vi "主界面.vi"() -> ()   [LabVIEW 2016]
uses:
  <vilib>/Hampel Software Engineering/HSE Logger/LogLevel.ctl
  <vilib>/Utility/miscctls.llb/LVPointTypeDef.ctl
  <vilib>/picture/picture.llb/imagedata.ctl
  <vilib>/Hampel Software Engineering/HSE Logger/Handler/FileHandler/FileHandler.lvclass
  C:/Program Files (x86)/National Instruments/LabVIEW 2016/vi.lib/Hampel Software Engineering/HSE Logger/Handler/Handler.lvclass
  <vilib>/Utility/config.llb/NI_LVConfig.lvlib
  <vilib>/Utility/LVLibp/NI_PackedLibraryUtility.lvlib
  update/update.lvlib
  <vilib>/Hampel Software Engineering/HSE Logger/hse-logger.lvlib
panel:
  in  "删除按钮":bool
  in  "添加按钮":bool
  in  "单选按钮":T1(radio)=enum."单选选项2"
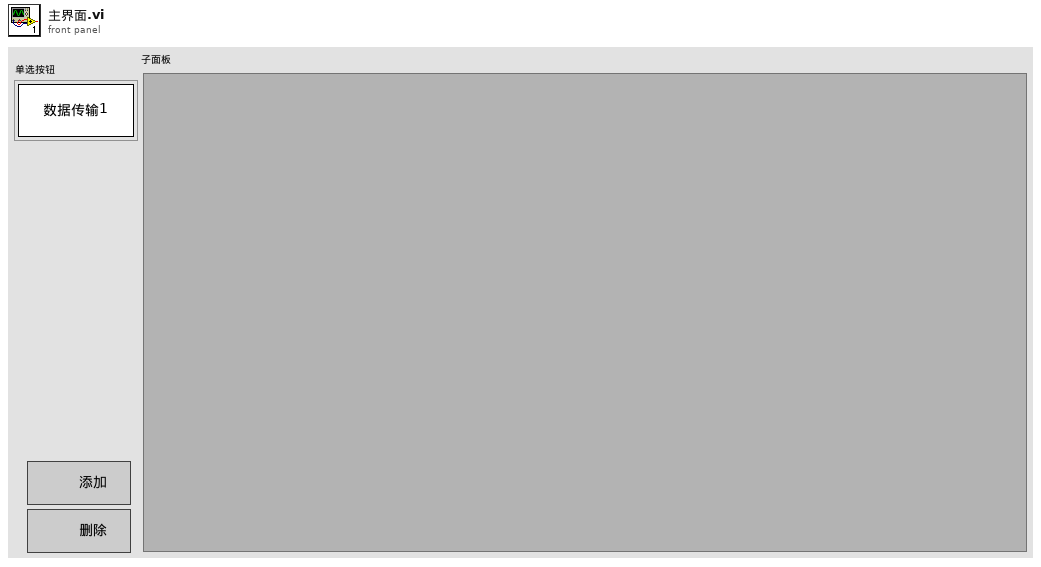
[diagram p1: front panel]
types:
  T1 = enum32{"数据传输1", "单选选项2", "单选选项3", "单选选项4", "单选选项5", "单选选项6"}
  T2 = typedef "hse-logger.lvlib/LogLevel.ctl" = enum16{"DEBUG", "INFO", "WARNING", "ERROR", "CRITICAL"}
  T3 = typedef "imagedata.ctl" = cluster{"image type":i32, "image depth":i32, "image":u8[], "mask":u8[], "colors":u32[], "Rectangle":cluster{"left":i16, "top":i16, "right":i16, "bottom":i16}}
  T4 = typedef "LVPointTypeDef.ctl" = cluster{"Horizontal":i16, "Vertical":i16}
  T5 = typedef "NI_LVConfig.lvlib/Config Data RefNum.ctl" = refnum<k1>
  T6 = enum32{"Bad", "Idle", "Run top level", "Running"}
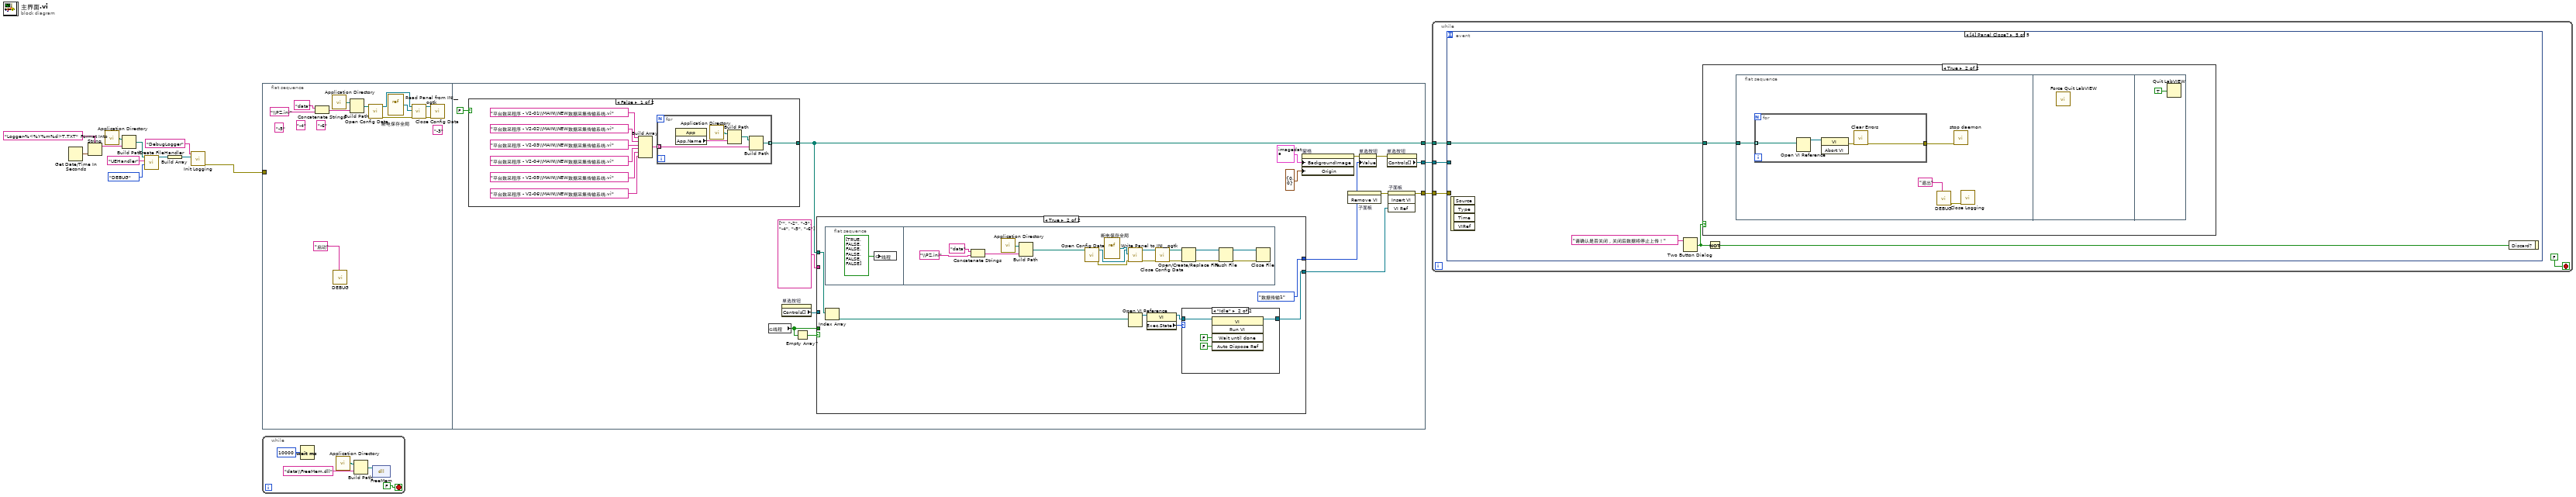
[diagram p0: block diagram]
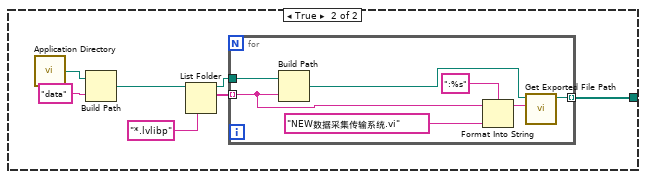
[diagram p2: hidden frame]
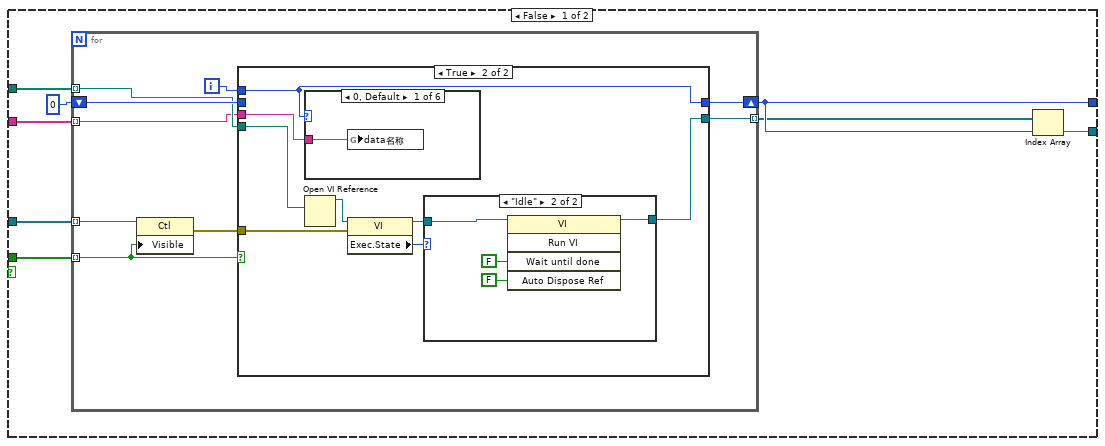
[diagram p3: hidden frame]
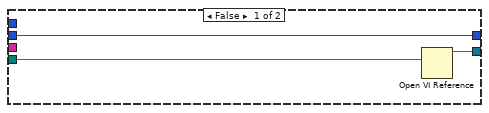
[diagram p4: hidden frame]
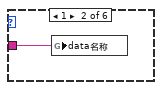
[diagram p5: hidden frame]
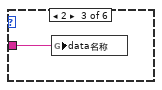
[diagram p6: hidden frame]
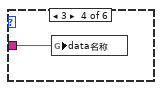
[diagram p7: hidden frame]
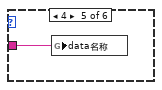
[diagram p8: hidden frame]
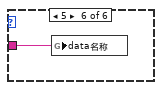
[diagram p9: hidden frame]
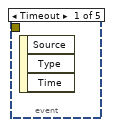
[diagram p12: hidden frame]
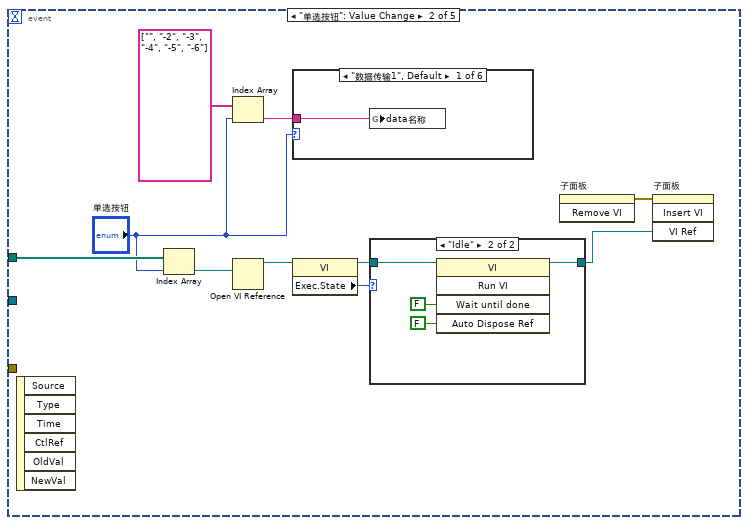
[diagram p13: hidden frame]
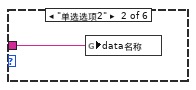
[diagram p14: hidden frame]
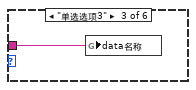
[diagram p15: hidden frame]
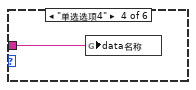
[diagram p16: hidden frame]
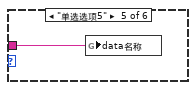
[diagram p17: hidden frame]
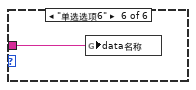
[diagram p18: hidden frame]
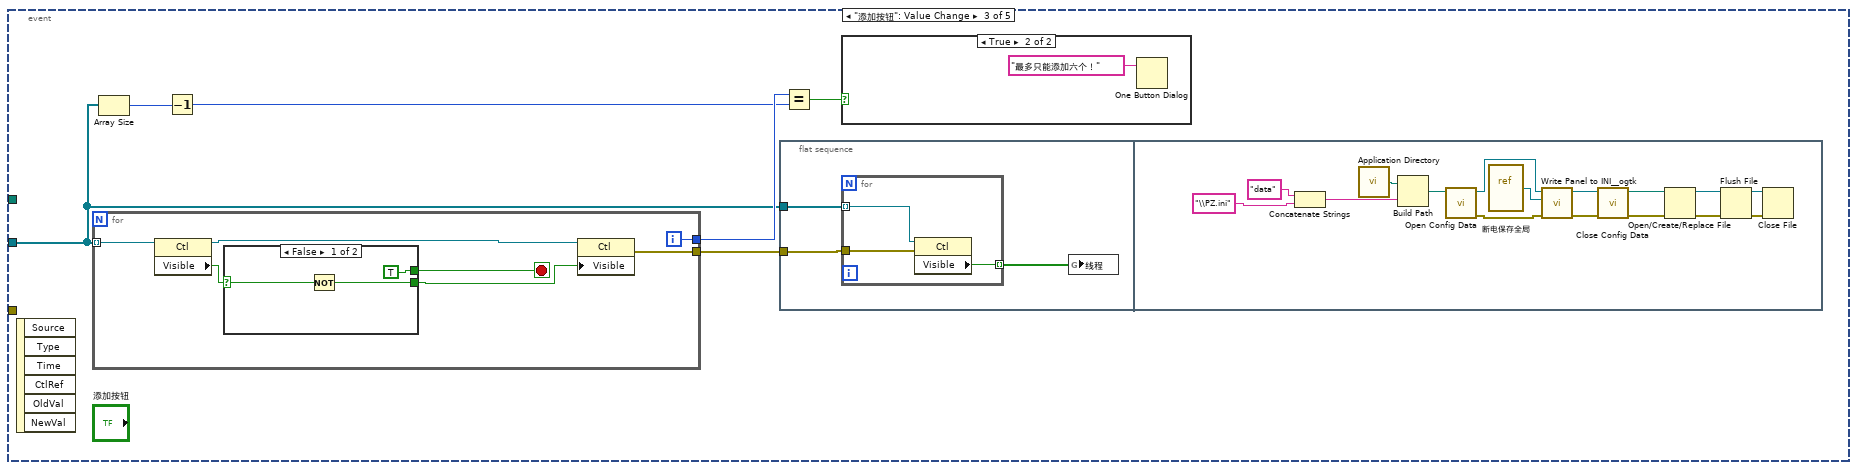
[diagram p20: hidden frame]
diagram:
  n1 = Get Date/Time In Seconds() -> (seconds since 1Jan1904=w4:timestamp)
  n2 = Format Into String(format string="Logger-%<%Y%m%d>T.TXT", w4) -> (resulting string=w5:string)  [unwired: 2 in, 1 out]
  n3 = call <vilib>:"Application Directory.vi"() -> ("Application Directory"=w7:path)
  n4 = Build Path(base path=w7, name or relative path=w5) -> (appended path=w6:path)
  n5 = call <vilib>:"Create FileHandler.vi"("Level"=LogLevel."DEBUG", "Name"="UEHandler", "Filepath"=w6) -> ("FileHandler out"=w9:refnum<class "FileHandler.lvclass">)  [unwired: 7 in, 1 out]
  n6 = Build Array(w9) -> (w10:refnum<class "FileHandler.lvclass">[])
  n7 = call <vilib>:"Init Logging.vi"("Handlers"=w10, "Name"="DebugLogger") -> ("error out"=w1:errorcluster)  [unwired: 9 in]
  n8 = flat-sequence {
    tunnel: w1 -> [_]
    tunnel: [w39] -> w14
    tunnel: [w38] -> w13
    tunnel: [w28] -> w12
    frame #0 {
      (unwired) "-6" ("data名称")
      (unwired) "-5" ("data名称")
      (unwired) "-4" ("data名称")
      (unwired) "-3" ("data名称")
      n9 = Concatenate Strings("data" ("名称或相对路径"), "\\PZ.ini" ("名称或相对路径")) -> (w24:string)
      n10 = call <vilib>:"Application Directory.vi"() -> ("Application Directory"=w20:path)
      n11 = call <vilib>:"DEBUG.vi"("Message"="启动") -> ()  [unwired: 10 in, 1 out]
      n12 = Build Path(base path=w20, name or relative path=w24) -> (appended path=w21:path)
      n13 = call <vilib>:"Open Config Data.vi"("configuration file path"=w21) -> ("error out"=w16:errorcluster, "refnum"=w17:T5)  [unwired: 8 in, 1 out]
      n14 = vi-ref "断电保存全局.vi"() -> (w18:refnum<vi>)
      n15 = call <userlib>:"Read Panel from INI__ogtk.vi"("error in (no error)"=w16, "VI ref"=w18, "refnum"=w17) -> ("error out"=w22:errorcluster, "refnum out"=w19:T5)  [unwired: 7 in]
      n16 = call <vilib>:"Close Config Data.vi"("error in (no error)"=w22, "refnum"=w19) -> ()  [unwired: 8 in, 2 out]
    }
    frame #1 {
      n17 = case shown="False" FALSE {
        tunnel: [w41 w54] -> w28
        frame False {
          n18 = Build Array("平台数采程序 - V2-01\\MAIN\\NEW数据采集传输系统.vi" ("名称或相对路径"), "平台数采程序 - V2-02\\MAIN\\NEW数据采集传输系统.vi" ("名称或相对路径"), "平台数采程序 - V2-03\\MAIN\\NEW数据采集传输系统.vi" ("名称或相对路径"), "平台数采程序 - V2-04\\MAIN\\NEW数据采集传输系统.vi" ("名称或相对路径"), "平台数采程序 - V2-05\\MAIN\\NEW数据采集传输系统.vi" ("名称或相对路径"), "平台数采程序 - V2-06\\MAIN\\NEW数据采集传输系统.vi" ("名称或相对路径")) -> (w48:string[])
          n19 = for {
            tunnel: w48 -> [w53] mode=indexing
            tunnel: [w52] -> w41 mode=indexing
            n20 = property class="App"() -> ("App.Name"=w51:string)  [unwired: 2 in, 2 out]
            n21 = call <vilib>:"Application Directory.vi"() -> ("Application Directory"=w50:path)
            n22 = Build Path(base path=w50, name or relative path=w51) -> (appended path=w49:path)
            n23 = Build Path(base path=w49, name or relative path=w53) -> (appended path=w52:path)
          }
        }
        frame True {
          n24 = call <vilib>:"Application Directory.vi"() -> ("Application Directory"=w57:path)
          n25 = Build Path(base path=w57, name or relative path="data" ("名称或相对路径")) -> (appended path=w59:path)
          n26 = List Folder(path=w59, pattern="*.lvlibp" ("类型")) -> (path out=w55:path, filenames=w56:string[])  [unwired: 2 in, 2 out]
          n27 = for {
            tunnel: w55 -> [w67]
            tunnel: w56 -> [w64] mode=indexing
            tunnel: [w61] -> w54 mode=indexing
            n28 = Build Path(base path=w67, name or relative path=w64) -> (appended path=w63:path)
            n29 = Format Into String(format string=":%s" ("格式字符串"), initial string=w64, "NEW数据采集传输系统.vi" ("输入 1")) -> (resulting string=w62:string)  [unwired: 1 in, 1 out]
            n30 = call <vilib>:"Get Exported File Path.vi"("qualified name"=w62, "packed library path"=w63) -> ("path"=w61:path)  [unwired: 8 in, 1 out]
          }
        }
      }
      n31 = global read "断电保存全局.vi" "线程"() -> (w33:bool[])
      n32 = property on="单选按钮" class="RadioBtnsControl (strict)"() -> ("Controls[]"=w32:refnum<vi>[])  [unwired: 2 in, 2 out]
      n33 = Empty Array?(array=w33) -> (empty?=w34:bool)
      n34 = case shown="True" w34 {
        tunnel: [w73 w111] -> w31
        tunnel: w33 -> [w75 _]
        tunnel: w32 -> [w74 _]
        tunnel: [w71 T1."数据传输1" ("单选按钮")] -> w30
        tunnel: w28 -> [w69 w108]
        tunnel: string[] ["", "-2", "-3", "-4", "-5", "-6"] -> [w68 _]
        frame False {
          n35 = for {
            tunnel: [w84] -> w70 mode=indexing
            tunnel: w75 -> [w83] mode=indexing
            tunnel: w74 -> [w82] mode=indexing
            shift-right: [w79] -> w71
            shift-left: 0 -> [w78]
            tunnel: w69 -> [w77] mode=indexing
            tunnel: w68 -> [w76] mode=indexing
            i -> [w80]
            n36 = property class="Ctl"(reference=w82, "Visible"=w83) -> (error out=w81:errorcluster)  [unwired: 1 in, 1 out]
            n37 = case shown="True" w83 {
              tunnel: [w86 w93] -> w84
              tunnel: w81 -> [_ w92]
              tunnel: w80 -> [_ w89]
              tunnel: [w87 w89] -> w79
              tunnel: w78 -> [w87 _]
              tunnel: w77 -> [w85 w90]
              tunnel: w76 -> [_ w88]
              frame False {
                n38 = Open VI Reference(vi path=w85) -> (vi reference=w86:refnum<vi>)  [unwired: 5 in, 1 out]
              }
              frame True {
                n39 = case shown="0, Default" w89 {
                  tunnel: w88 -> [w96 w97 w98 w99 w100 w101]
                  frame 0, Default {
                    n40 = global write "断电保存全局.vi" "data名称"(w96) -> ()
                  }
                  frame 1 {
                    n41 = global write "断电保存全局.vi" "data名称"(w97) -> ()
                  }
                  frame 2 {
                    n42 = global write "断电保存全局.vi" "data名称"(w98) -> ()
                  }
                  frame 3 {
                    n43 = global write "断电保存全局.vi" "data名称"(w99) -> ()
                  }
                  frame 4 {
                    n44 = global write "断电保存全局.vi" "data名称"(w100) -> ()
                  }
                  frame 5 {
                    n45 = global write "断电保存全局.vi" "data名称"(w101) -> ()
                  }
                }
                n46 = Open VI Reference(vi path=w90) -> (vi reference=w91:refnum<vi>)  [unwired: 5 in, 1 out]
                n47 = property class="VI"(reference=w91, error in=w92) -> (reference out=w95:refnum<vi>, "Exec.State"=w94:T6)  [unwired: 1 out]
                n48 = case shown="\"Idle\"" w94 {
                  tunnel: w95 -> [w102 w104]
                  tunnel: [w102 w103] -> w93
                  frame "Bad", Default {
                  }
                  frame "Idle" {
                    n49 = invoke class="VI" method="Run VI"(reference=w104, "Wait until done"=FALSE ("结束前等待"), "Auto Dispose Ref"=FALSE ("自动销毁引用")) -> (reference out=w103:refnum<vi>)  [unwired: 2 in, 4 out]
                  }
                }
              }
            }
          }
          n50 = Index Array(array=w70, index=w71) -> (element=w73:refnum<vi>)
        }
        frame True {
          n51 = flat-sequence {
            frame #0 {
              n52 = global write "断电保存全局.vi" "线程"(bool[] [TRUE, FALSE, FALSE, FALSE, FALSE, FALSE] ("线程")) -> ()
            }
            frame #1 {
              n53 = Concatenate Strings("data" ("名称或相对路径"), "\\PZ.ini" ("名称或相对路径")) -> (w116:string)
              n54 = call <vilib>:"Application Directory.vi"() -> ("Application Directory"=w118:path)
              n55 = Build Path(base path=w118, name or relative path=w116) -> (appended path=w119:path)
              n56 = call <vilib>:"Open Config Data.vi"("configuration file path"=w119) -> ("error out"=w123:errorcluster, "refnum"=w120:T5)  [unwired: 8 in, 1 out]
              n57 = vi-ref "断电保存全局.vi"() -> (w121:refnum<vi>)
              n58 = call <userlib>:"Write Panel to INI__ogtk.vi"("error in (no error)"=w123, "VI ref"=w121, "refnum"=w120) -> ("error out"=w124:errorcluster, "refnum out"=w122:T5)  [unwired: 7 in]
              n59 = call <vilib>:"Close Config Data.vi"("error in (no error)"=w124, "refnum"=w122) -> ("error out"=w129:errorcluster, "file path"=w130:path)  [unwired: 8 in]
              n60 = Open/Create/Replace File(file path (use dialog)=w130, error in=w129) -> (refnum out=w126:refnum<file>, error out=w125:errorcluster)  [unwired: 4 in, 1 out]
              n61 = Flush File(refnum=w126, error in=w125) -> (refnum out=w127:refnum<file>, error out=w128:errorcluster)
              n62 = Close File(refnum=w127, error in=w128) -> ()  [unwired: 2 out]
            }
          }
          n63 = Index Array(array=w108) -> (element=w107:path)  [unwired: 1 in]
          n64 = Open VI Reference(vi path=w107) -> (vi reference=w109:refnum<vi>)  [unwired: 5 in, 1 out]
          n65 = property class="VI"(reference=w109) -> (reference out=w113:refnum<vi>, "Exec.State"=w112:T6)  [unwired: 1 in, 1 out]
          n66 = case shown="\"Idle\"" w112 {
            tunnel: w113 -> [w131 w133]
            tunnel: [w131 w132] -> w111
            frame "Bad", Default {
            }
            frame "Idle" {
              n67 = invoke class="VI" method="Run VI"(reference=w133, "Wait until done"=FALSE ("结束前等待"), "Auto Dispose Ref"=FALSE ("自动销毁引用")) -> (reference out=w132:refnum<vi>)  [unwired: 2 in, 4 out]
            }
          }
        }
      }
      n68 = property on="窗格" class="Pane"("BackgroundImage"=T3 {"image type"=0, "image depth"=24, "image"=array[12288000 elements], "mask"=[], "colors"=[], "Rectangle"={"left"=0, "top"=0, "right"=2560, "bottom"=1600}} ("image data"), "Origin"=T4 {"Horizontal"=0, "Vertical"=0} ("原点")) -> (error out=w35:errorcluster)  [unwired: 2 in, 1 out]
      n69 = invoke on="子面板" class="SubPnl" method="Remove VI"() -> (error out=w40:errorcluster)  [unwired: 3 in, 2 out]
      n70 = property on="单选按钮" class="RadioBtnsControl (strict)"(error in=w35, "Value"=w30) -> (error out=w37:errorcluster)  [unwired: 1 in, 1 out]
      n71 = property on="单选按钮" class="RadioBtnsControl (strict)"(error in=w37) -> ("Controls[]"=w38:refnum<vi>[])  [unwired: 1 in, 2 out]
      n72 = invoke on="子面板" class="SubPnl" method="Insert VI"(error in=w40, "VI Ref"=w31) -> (error out=w39:errorcluster)  [unwired: 2 in, 3 out]
    }
  }
  n73 = while {
    stop <- FALSE stop-if-true
    n74 = Wait (ms)(milliseconds to wait=u32 10000 ("等待时间（毫秒）")) -> ()  [unwired: 1 out]
    n75 = call <vilib>:"Application Directory.vi"() -> ("Application Directory"=w137:path)
    n76 = Build Path(base path=w137, name or relative path="data\\FreeMem.dll" ("名称或相对路径")) -> (appended path=w136:path)
    n77 = dll-call lib="PTH2Habs F\tgitkrakenCC数据传输套壳多开-V2.1dataFreeMem.dll" fn="FreeMem"(path in=w136) -> ()  [unwired: 3 in, 2 out]
  }
  n78 = while {
    tunnel: w14 -> [w142]
    tunnel: w13 -> [w143]
    tunnel: w12 -> [w141]
    stop <- FALSE stop-if-true
    n79 = event shown="[4] Panel Close?" {
      selector: _ -> [_ _ _ _ _]
      dyn-events: _ -> [_ _ _ _ _]
      timeout: _ -> [_ _ _ _ _]
      tunnel: w143 -> [_ _ w166 w208 _]
      tunnel: w142 -> [_ _ _ w214 _]
      tunnel: w141 -> [_ w149 _ w207 w264]
      event Timeout {
        n80 = event-data() -> ()  [unwired: 1 in, 3 out]
      }
      event "单选按钮": Value Change {
        n81 = event-data() -> ()  [unwired: 1 in, 6 out]
        n82 = Index Array(array=w149, index="单选按钮") -> (element=w148:path)
        n83 = Index Array(array=string[] ["", "-2", "-3", "-4", "-5", "-6"], index="单选按钮") -> (element=w145:string)
        n84 = Open VI Reference(vi path=w148) -> (vi reference=w150:refnum<vi>)  [unwired: 5 in, 1 out]
        n85 = case shown="\"数据传输1\", Default" "单选按钮" {
          tunnel: w145 -> [w155 w156 w157 w158 w159 w160]
          frame "数据传输1", Default {
            n86 = global write "断电保存全局.vi" "data名称"(w155) -> ()
          }
          frame "单选选项2" {
            n87 = global write "断电保存全局.vi" "data名称"(w156) -> ()
          }
          frame "单选选项3" {
            n88 = global write "断电保存全局.vi" "data名称"(w157) -> ()
          }
          frame "单选选项4" {
            n89 = global write "断电保存全局.vi" "data名称"(w158) -> ()
          }
          frame "单选选项5" {
            n90 = global write "断电保存全局.vi" "data名称"(w159) -> ()
          }
          frame "单选选项6" {
            n91 = global write "断电保存全局.vi" "data名称"(w160) -> ()
          }
        }
        n92 = property class="VI"(reference=w150) -> (reference out=w153:refnum<vi>, "Exec.State"=w154:T6)  [unwired: 1 in, 1 out]
        n93 = case shown="\"Idle\"" w154 {
          tunnel: w153 -> [w161 w163]
          tunnel: [w161 w162] -> w151
          frame "Bad", Default {
          }
          frame "Idle" {
            n94 = invoke class="VI" method="Run VI"(reference=w163, "Wait until done"=FALSE ("结束前等待"), "Auto Dispose Ref"=FALSE ("自动销毁引用")) -> (reference out=w162:refnum<vi>)  [unwired: 2 in, 4 out]
          }
        }
        n95 = invoke on="子面板" class="SubPnl" method="Remove VI"() -> (error out=w152:errorcluster)  [unwired: 3 in, 2 out]
        n96 = invoke on="子面板" class="SubPnl" method="Insert VI"(error in=w152, "VI Ref"=w151) -> ()  [unwired: 2 in, 4 out]
      }
      event "添加按钮": Value Change {
        n97 = event-data() -> ()  [unwired: 1 in, 6 out]
        n98 = for {
          tunnel: w166 -> [w201] mode=indexing
          tunnel: [w196] -> w170
          tunnel: [w195] -> w167
          i -> [w196]
          stop <- w197 stop-if-true
          n99 = property class="Ctl"(reference=w201) -> (reference out=w199:refnum<vi>, "Visible"=w200:bool)  [unwired: 1 in, 1 out]
          n100 = case shown="False" w200 {
            selector: w200 -> [w204 w206]
            tunnel: [w203 w206] -> w198
            tunnel: [TRUE FALSE] -> w197
            frame False {
              n101 = Not(x=w204) -> (.not. x?=w203:bool)
            }
            frame True {
            }
          }
          n102 = property class="Ctl"(reference=w199, "Visible"=w198) -> (error out=w195:errorcluster)  [unwired: 1 in, 1 out]
        }
        n103 = Array Size(array=w166) -> (size(s)=w171:i32)
        n104 = Decrement(x=w171) -> (x-1=w169:i32)
        n105 = flat-sequence {
          tunnel: w167 -> [w173]
          tunnel: w166 -> [w172]
          frame #0 {
            n106 = for {
              tunnel: w172 -> [w177] mode=indexing
              tunnel: [w176] -> w174 mode=indexing
              tunnel: w173 -> [w175]
              n107 = property class="Ctl"(reference=w177, error in=w175) -> ("Visible"=w176:bool)  [unwired: 2 out]
            }
            n108 = global write "断电保存全局.vi" "线程"(w174) -> ()
          }
          frame #1 {
            n109 = Concatenate Strings("data" ("名称或相对路径"), "\\PZ.ini" ("名称或相对路径")) -> (w179:string)
            n110 = call <vilib>:"Application Directory.vi"() -> ("Application Directory"=w181:path)
            n111 = Build Path(base path=w181, name or relative path=w179) -> (appended path=w182:path)
            n112 = call <vilib>:"Open Config Data.vi"("configuration file path"=w182) -> ("error out"=w186:errorcluster, "refnum"=w183:T5)  [unwired: 8 in, 1 out]
            n113 = vi-ref "断电保存全局.vi"() -> (w184:refnum<vi>)
            n114 = call <userlib>:"Write Panel to INI__ogtk.vi"("error in (no error)"=w186, "VI ref"=w184, "refnum"=w183) -> ("error out"=w187:errorcluster, "refnum out"=w185:T5)  [unwired: 7 in]
            n115 = call <vilib>:"Close Config Data.vi"("error in (no error)"=w187, "refnum"=w185) -> ("error out"=w192:errorcluster, "file path"=w193:path)  [unwired: 8 in]
            n116 = Open/Create/Replace File(file path (use dialog)=w193, error in=w192) -> (refnum out=w189:refnum<file>, error out=w188:errorcluster)  [unwired: 4 in, 1 out]
            n117 = Flush File(refnum=w189, error in=w188) -> (refnum out=w190:refnum<file>, error out=w191:errorcluster)
            n118 = Close File(refnum=w190, error in=w191) -> ()  [unwired: 2 out]
          }
        }
        n119 = Equal?(x=w170, y=w169) -> (x = y?=w168:bool)
        n120 = case shown="True" w168 {
          frame False {
          }
          frame True {
            n121 = One Button Dialog(message="最多只能添加六个！" ("消息")) -> ()  [unwired: 1 in, 1 out]
          }
        }
      }
      event "删除按钮": Value Change {
        n122 = event-data() -> ()  [unwired: 1 in, 6 out]
        n123 = for {
          tunnel: w208 -> [w260] mode=indexing
          shift-right: [w258] -> w212
          shift-left: 0 -> [w259]
          n124 = property class="Ctl"(reference=w260) -> ("Visible"=w257:bool)  [unwired: 1 in, 2 out]
          n125 = case shown="True" w257 {
            tunnel: w259 -> [w261 w263]
            tunnel: [w261 w262] -> w258
            frame False {
            }
            frame True {
              n126 = Increment(x=w263) -> (x+1=w262:i32)
            }
          }
        }
        n127 = Greater?(x=w212, y=1) -> (0:w210:bool)
        n128 = case shown="True" w210 {
          tunnel: w214 -> [_ w251]
          tunnel: w208 -> [_ w242]
          tunnel: [_ w241] -> w209
          tunnel: w207 -> [_ w239]
          frame False {
            n129 = One Button Dialog(message="已经最小单元，无法删除！" ("消息")) -> ()  [unwired: 1 in, 1 out]
          }
          frame True {
            n130 = invoke on="子面板" class="SubPnl" method="Remove VI"(error in=w251) -> (error out=w248:errorcluster)  [unwired: 2 in, 2 out]
            n131 = property on="单选按钮" class="RadioBtnsControl (strict)"(error in=w248) -> (error out=w246:errorcluster, "Value"=w247:T1)  [unwired: 1 in, 1 out]
            n132 = Index Array(array=w239, index=w247) -> (element=w238:path)
            n133 = Open VI Reference(vi path=w238) -> (vi reference=w240:refnum<vi>)  [unwired: 5 in, 1 out]
            n134 = invoke class="VI" method="Abort VI"(reference=w240, error in=w246) -> (error out=w245:errorcluster)  [unwired: 1 in, 2 out]
            n135 = Index Array(array=w242, index=w247) -> (element=w250:refnum<vi>)
            n136 = property class="Ctl"(reference=w250, error in=w245, "Visible"=FALSE ("可见")) -> (error out=w243:errorcluster)  [unwired: 1 out]
            n137 = for {
              tunnel: w242 -> [w256] mode=indexing
              tunnel: [w254] -> w244
              tunnel: w243 -> [w253]
              tunnel: [w252] -> w241
              i -> [w254]
              stop <- w255 stop-if-true
              n138 = property class="Ctl"(reference=w256, error in=w253) -> (error out=w252:errorcluster, "Visible"=w255:bool)  [unwired: 1 out]
            }
            n139 = property on="单选按钮" class="RadioBtnsControl (strict)"(error in=w241, "Val(Sgnl)"=w244) -> ()  [unwired: 1 in, 2 out]
          }
        }
        n140 = flat-sequence {
          tunnel: w209 -> [w216]
          tunnel: w208 -> [w215]
          frame #0 {
            n141 = for {
              tunnel: w215 -> [w220] mode=indexing
              tunnel: [w219] -> w217 mode=indexing
              tunnel: w216 -> [w218]
              n142 = property class="Ctl"(reference=w220, error in=w218) -> ("Visible"=w219:bool)  [unwired: 2 out]
            }
            n143 = global write "断电保存全局.vi" "线程"(w217) -> ()
          }
          frame #1 {
            n144 = Concatenate Strings("data" ("名称或相对路径"), "\\PZ.ini" ("名称或相对路径")) -> (w222:string)
            n145 = call <vilib>:"Application Directory.vi"() -> ("Application Directory"=w224:path)
            n146 = Build Path(base path=w224, name or relative path=w222) -> (appended path=w225:path)
            n147 = call <vilib>:"Open Config Data.vi"("configuration file path"=w225) -> ("error out"=w229:errorcluster, "refnum"=w226:T5)  [unwired: 8 in, 1 out]
            n148 = vi-ref "断电保存全局.vi"() -> (w227:refnum<vi>)
            n149 = call <userlib>:"Write Panel to INI__ogtk.vi"("error in (no error)"=w229, "VI ref"=w227, "refnum"=w226) -> ("error out"=w230:errorcluster, "refnum out"=w228:T5)  [unwired: 7 in]
            n150 = call <vilib>:"Close Config Data.vi"("error in (no error)"=w230, "refnum"=w228) -> ("error out"=w235:errorcluster, "file path"=w236:path)  [unwired: 8 in]
            n151 = Open/Create/Replace File(file path (use dialog)=w236, error in=w235) -> (refnum out=w232:refnum<file>, error out=w231:errorcluster)  [unwired: 4 in, 1 out]
            n152 = Flush File(refnum=w232, error in=w231) -> (refnum out=w233:refnum<file>, error out=w234:errorcluster)
            n153 = Close File(refnum=w233, error in=w234) -> ()  [unwired: 2 out]
          }
        }
      }
      event Panel Close? {
        n154 = event-data() -> ()  [unwired: 1 in, 4 out]
        n155 = Two Button Dialog(message="请确认是否关闭，关闭后数据将停止上传！" ("消息")) -> (T button?=w265:bool)  [unwired: 2 in]
        n156 = case shown="True" w265 {
          tunnel: w264 -> [_ w268]
          frame False {
          }
          frame True {
            n157 = flat-sequence {
              tunnel: w268 -> [w272]
              frame #0 {
                n158 = for {
                  tunnel: w272 -> [w274] mode=indexing
                  tunnel: [w273] -> w271
                  n159 = Open VI Reference(vi path=w274) -> (vi reference=w275:refnum<vi>)  [unwired: 5 in, 1 out]
                  n160 = invoke class="VI" method="Abort VI"(reference=w275) -> (error out=w276:errorcluster)  [unwired: 2 in, 2 out]
                  n161 = call <vilib>:"Clear Errors.vi"("error in (no error)"=w276) -> ("error out"=w273:errorcluster)  [unwired: 5 in, 1 out]
                }
                n162 = call <vilib>:"DEBUG.vi"("Message"="退出") -> ("error out"=w269:errorcluster)  [unwired: 10 in]
                n163 = call "stop daemon.vi"("error in (no error)"=w271) -> ()  [unwired: 10 in, 1 out]
                n164 = call <vilib>:"Close Logging.vi"("error in"=w269) -> ()  [unwired: 10 in, 1 out]
              }
              frame #1 {
                n165 = call "Force Quit LabVIEW.vi"() -> ()  [unwired: 10 in, 2 out]
              }
              frame #2 {
                n166 = Quit LabVIEW(quit? (T)=TRUE ("退出？(T)")) -> ()
              }
            }
          }
        }
        n167 = Not(x=w265) -> (.not. x?=w266:bool)
        n168 = event-data("Discard?"=w266) -> ()  [unwired: 1 in, 1 out]
      }
    }
  }
